vi "RSNRPZ Sensors Info Header.vi"(7 "Array Size (100)":i32=100, 8 "error in (no error)":errorcluster, 9 "Parameter Number (0)":i32, 10 "Channel (1)":i32=1, 11 "VISA session":refnum<visa-resource-name> caption="VISA resource name") -> (0 "error out":errorcluster, 2 "Header":string, 3 "dup VISA session":refnum<visa-resource-name> caption="VISA resource name")   [LabVIEW 2010]
doc: "This function returns header and value of a certain line within the result of the SYST:INFO? query \nSYST:INFO? query returns an array of strings, where every line denotes a certain sensor parameter.\n-- For example, SYST:INFO? could return \n      Manufacturer:Rohde & Schwarz \n      Type:NRP-Z85 \n      Stock Number:1411.7501.02 \n      Serial:900003 \n      HWVersion:000000000 \n      HWVariant:000000000 \n      SW Build:01.37 \n      FPGA Build:TS:28;SC:22;ST:22 \n      Technology:Diode \n      Function:Power Terminating \n      MinPower:1e-09 \n      MaxPower:0.1 \n      MinFreq:5e+07 \n      MaxFreq:4e+10 \n      :: \n      :: \n           \nIn this example a call of rsnrpz_chan_infoHeader() with a parameterNb = 6 would return the 6th line, which contains the sensor Firmware version (--> \"SW Build:01.37\" in this case).\n\nRemote-control command(s):\nSYST:INFO?"
uses:
  rsnrpz_32.dll
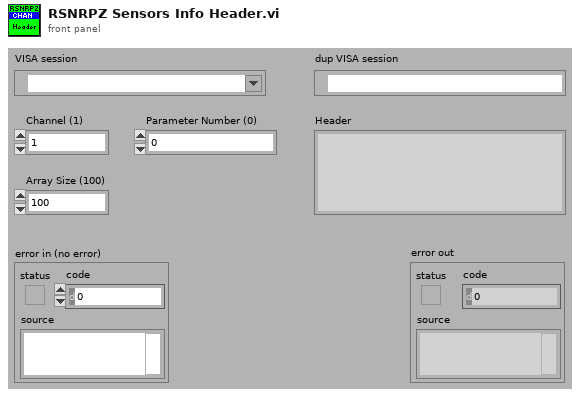
[diagram p1: front panel]
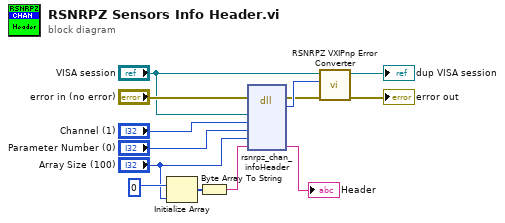
[diagram p0: block diagram]
diagram:
  n1 = Initialize Array(u8 0, "Array Size (100)") -> (w12:u8[])
  n2 = Byte Array To String(unsigned byte array=w12) -> (string=w8:string)
  n3 = dll-call lib="rsnrpz_32.dll" fn="rsnrpz_chan_infoHeader"(error in="error in (no error)", "Instrument Handle"="VISA session", "Channel"="Channel (1)", "Parameter Number"="Parameter Number (0)", "Array Size"="Array Size (100)", "Header"=w8) -> (error out=w5:errorcluster, "Status"=w11:i32, "Header"=→"Header":string)  [unwired: 6 in, 1 out]
  n4 = call <instrlib>:"RSNRPZ VXIPnp Error Converter.vi"("error in"=w5, "VXIPnp error code"=w11, "VISA session"="VISA session") -> ("error out"=→"error out":errorcluster, "dup VISA session"=→"dup VISA session":refnum<visa-resource-name>)  [unwired: 7 in]
